vi "HGF_DSCMonitor.appendData2Variant.vi"(2 "initData":variant, 3 "timeout":i32, 5 "error in (no error)":errorcluster) -> (16 "dup initData":variant, 19 "error out":errorcluster)   [LabVIEW 2012, in "HGF_DSC.lvlib" / "HGF_DSCMonitor.lvclass"]
uses:
  HGF_DSCMonitor.lvclass
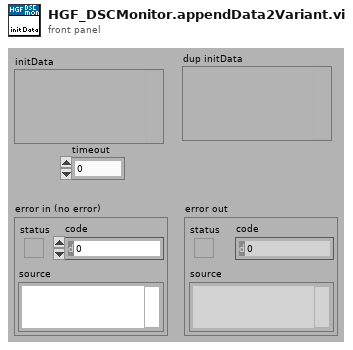
[diagram p1: front panel]
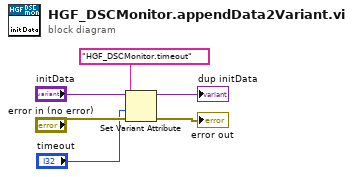
[diagram p0: block diagram]
diagram:
  n1 = Set Variant Attribute(Variant="initData", name="HGF_DSCMonitor.timeout", value="timeout", error in="error in (no error)") -> (Variant out=→"dup initData":variant, error out=→"error out":errorcluster)  [unwired: 1 out]
